vi "Tunnel Speed Ch Names.vi"(4 "Rig Name":string) -> (0 "Calib Tweak":string, 1 "Dem Voltage":string, 2 "Dem Velocity":string)   [LabVIEW 2022 SP3]
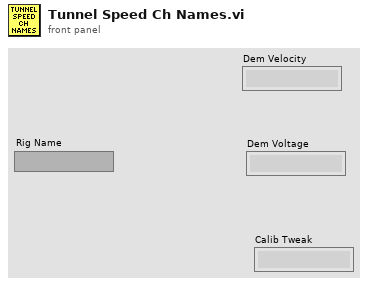
[diagram p1: front panel]
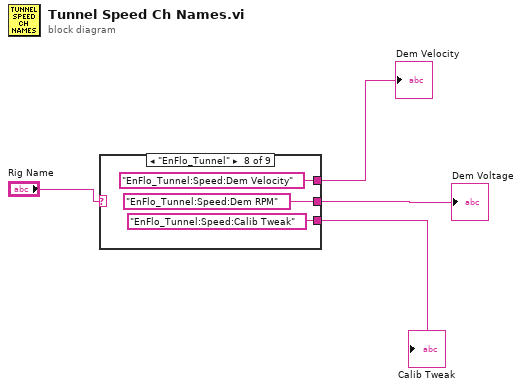
[diagram p0: block diagram]
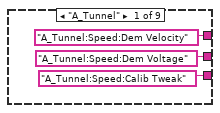
[diagram p2: hidden frame]
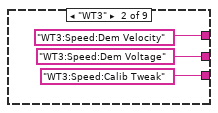
[diagram p3: hidden frame]
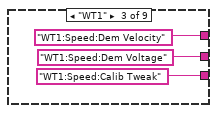
[diagram p4: hidden frame]
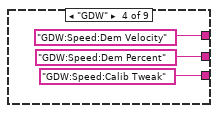
[diagram p5: hidden frame]
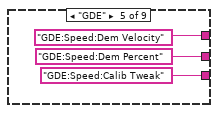
[diagram p6: hidden frame]
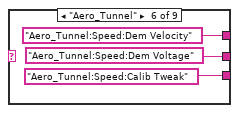
[diagram p7: hidden frame]
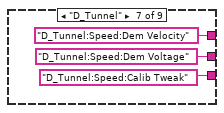
[diagram p8: hidden frame]
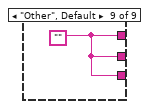
[diagram p9: hidden frame]
diagram:
  n1 = case shown="\"EnFlo_Tunnel\"" "Rig Name" {
    tunnel: ["A_Tunnel:Speed:Dem Velocity" "WT3:Speed:Dem Velocity" "WT1:Speed:Dem Velocity" "GDW:Speed:Dem Velocity" "GDE:Speed:Dem Velocity" "Aero_Tunnel:Speed:Dem Velocity" "D_Tunnel:Speed:Dem Velocity" "EnFlo_Tunnel:Speed:Dem Velocity" w29] -> w3
    tunnel: ["A_Tunnel:Speed:Dem Voltage" "WT3:Speed:Dem Voltage" "WT1:Speed:Dem Voltage" "GDW:Speed:Dem Percent" "GDE:Speed:Dem Percent" "Aero_Tunnel:Speed:Dem Voltage" "D_Tunnel:Speed:Dem Voltage" "EnFlo_Tunnel:Speed:Dem RPM" w29] -> w2
    tunnel: ["A_Tunnel:Speed:Calib Tweak" "WT3:Speed:Calib Tweak" "WT1:Speed:Calib Tweak" "GDW:Speed:Calib Tweak" "GDE:Speed:Calib Tweak" "Aero_Tunnel:Speed:Calib Tweak" "D_Tunnel:Speed:Calib Tweak" "EnFlo_Tunnel:Speed:Calib Tweak" w29] -> w1
    frame "A_Tunnel" {
    }
    frame "WT3" {
    }
    frame "WT1" {
    }
    frame "GDW" {
    }
    frame "GDE" {
    }
    frame "Aero_Tunnel" {
    }
    frame "D_Tunnel" {
    }
    frame "EnFlo_Tunnel" {
    }
    frame "Other", Default {
      w29 = ""
    }
  }
  "Dem Velocity" <- w3
  "Dem Voltage" <- w2
  "Calib Tweak" <- w1
